vi "Open Demosaicker.vi"(8 "error in (no error)":errorcluster) -> (0 "error out":errorcluster, 3 "Demosaicker reference":refnum<k24>)   [LabVIEW 2022 SP3]
uses:
  I:/.shortcut-targets-by-id/1riZacJd_1_jmKfGgrjDuP7KcecvMS3i2/Xiao research group/Programs/XYZRecorrection/Scientific Camera Interfaces/SDK/DotNet Toolkit/dlls/Managed_64_lib/Thorlabs.TSI.Demosaicker.dll
  SDK/DotNet Toolkit/dlls/Managed_64_lib/Thorlabs.TSI.Demosaicker.dll
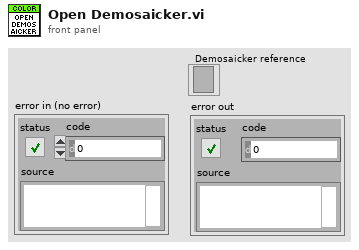
[diagram p1: front panel]
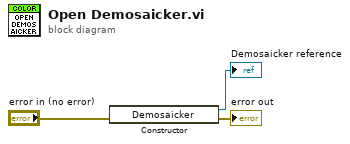
[diagram p0: block diagram]
diagram:
  n1 = constructor class="Demosaicker"(error in="error in (no error)") -> (reference out=→"Demosaicker reference":refnum<k24>, error out=→"error out":errorcluster)  [unwired: 2 in, 1 out]
